vi "CR-字符图片显示.vi"(0 "Image in":T2(plugin-control), 7 "是否检测到字符串":bool, 9 "String (OCR/OCV 1)":string, 11 "error in (no error)":errorcluster caption="错误输入（无错误）", 12 "ROI Descriptor":T1 {"Contours"."Type" items=["No Selection", "Point", "Line", "Rectangle", "Oval", "Polygon", "Freehand Region", "Annulus", "Unused2", "Unused3", "Broken Line", "Freehand Line", "Rotated Rectangle"]}) -> (4 "Image out":T2(plugin-control), 15 "error out":errorcluster caption="错误输出")   [LabVIEW 2017]
panel:
  out "字符串":string
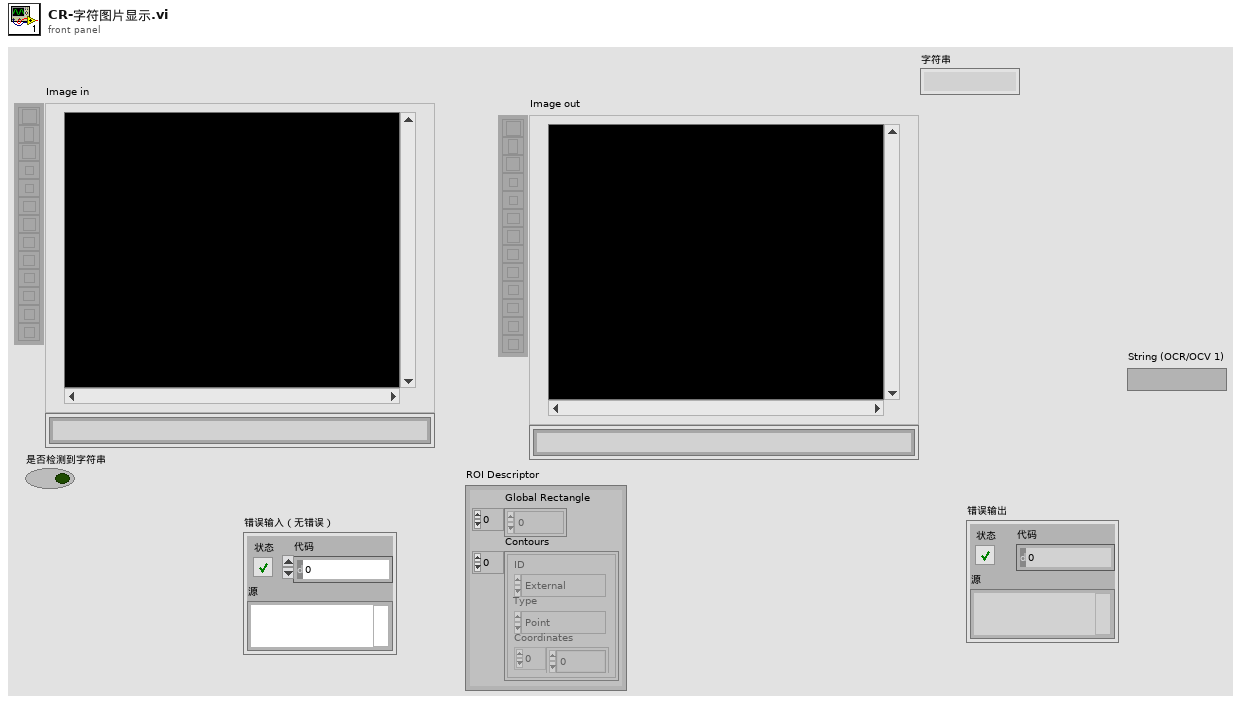
[diagram p1: front panel]
types:
  T1 = typedef "ROI Descriptor" = cluster{"Global Rectangle":i32[], "Contours":cluster{"ID":enum32{"External", "Internal"}, "Type":u32, "Coordinates":i32[]}[]}
  T2 = typedef "IMAQ Image.ctl" = refnum<image>
  T3 = cluster{"Desired Font (Application)":enum16{"User-specified Font", "Application Font", "System Font", "Dialog Font"}, "[User-specified Font]":cluster{"Font Name":string, "Size":i16, "Strikeout?":bool, "Italic?":bool, "Underline?":bool, "Outline?":bool, "Shadow?":bool, "Bold?":bool, "Rotation Angle":dbl}, "Horizontal Alignment":i16, "Vertical Alignment":i16}
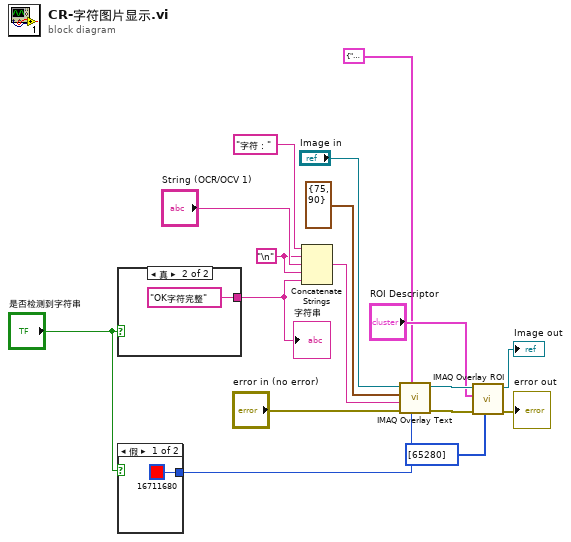
[diagram p0: block diagram]
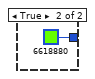
[diagram p2: hidden frame]
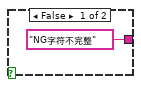
[diagram p3: hidden frame]
diagram:
  w10 = "\n"
  n1 = case shown="真" "是否检测到字符串" {
    tunnel: ["NG字符不完整" "OK字符完整"] -> w9
    frame False {
    }
    frame True {
    }
  }
  "字符串" <- w9
  n2 = case shown="假" "是否检测到字符串" {
    tunnel: [u32 16711680 ("Text Color (black)") u32 6618880 ("Text Color (black)")] -> w15
    frame False {
    }
    frame True {
    }
  }
  n3 = Concatenate Strings("字符：" ("字符串"), w10, "String (OCR/OCV 1)", w10, w9) -> (w17:string)
  n4 = call "IMAQ Overlay Text"("Text Color (black)"=w15, "Font, Size & Style"=T3 {"Desired Font (Application)"=enum."User-specified Font", "[User-specified Font]"={"Font Name"="", "Size"=50, "Strikeout?"=FALSE, "Italic?"=FALSE, "Underline?"=FALSE, "Outline?"=FALSE, "Shadow?"=TRUE, "Bold?"=TRUE, "Rotation Angle"=0.0}, "Horizontal Alignment"=0, "Vertical Alignment"=0}, "error in (no error)"="error in (no error)", "String"=w17, "Origin"=cluster{"X":i32, "Y":i32} {"X"=75, "Y"=90}, "Image"="Image in") -> ("error out"=w2:errorcluster, "Image Out"=w12:T2)  [unwired: 4 in]
  n5 = call "IMAQ Overlay ROI"("Colors (Green)"=u32[] [65280], "error in (no error)"=w2, "ROI Descriptor"="ROI Descriptor", "Image"=w12) -> ("error out"=→"error out":errorcluster, "Image Out"=→"Image out":T2)  [unwired: 6 in]
